vi "Unit Test.vi"() -> ()   [LabVIEW 2019, in "Test.lvlib"]
uses:
  Test.lvlib
  User Event/Controls/UE Abort Action.ctl
  Syringe Pump/NE-500/NE-500.lvlib
  Selection Valve/IDEX/IDEX.lvlib
  LED/LED.lvlib
  IO/sbRIO9623/sbRIO9623.lvlib
  Fluidic Process/Fluidic Process.lvlib
panel:
  in  "UI":bool
  out "Syringe Pump":bool
  out "Selection Valve":bool
  out "LED":bool
  out "I/O":bool
  in  "Open":bool
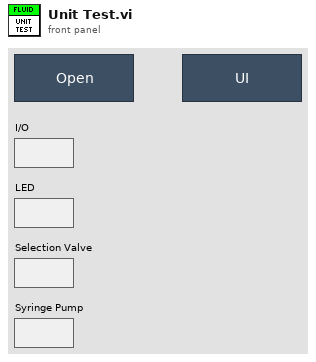
[diagram p1: front panel]
types:
  T1 = typedef "UE Abort Action.ctl" = enum16{"Create", "Get", "Destroy"}
  T2 = typedef "sbRIO9623.lvlib/SEQ Data.ctl" = cluster{"Lid Sensor 1":bool, "Lid Sensor 2":bool, "Laser Interlock":bool, "Buffer Tank":bool, "Wash Tank":bool, "Waste Tank":bool, "SiPM 1":fxp<+,20,5>, "SiPM 2":fxp<+,20,5>, "Initialize Success?":bool, "VI Refnum":refnum<vi>}
  T3 = typedef "LED.lvlib/SEQ Data.ctl" = cluster{"Initialize Sucess?":bool, "BL2 Regulator":dbl, "BL1 Regulator":dbl, "Blood Sensor 1":dbl, "Blood Sensor 2":dbl, "Air Pressure Sensor":dbl, "Force Snesor 1":u32, "Force Snesor 2":u32, "VI Refnum":refnum<vi>}
  T4 = typedef "IDEX.lvlib/SEQ Data.ctl" = cluster{"Position":string, "Initialize Done?":bool, "VI Refnum":refnum<vi>}
  T5 = typedef "NE-500.lvlib/SEQ Data.ctl" = cluster{"Status":string, "Initialize Done?":bool, "VI Refnum":refnum<vi>}
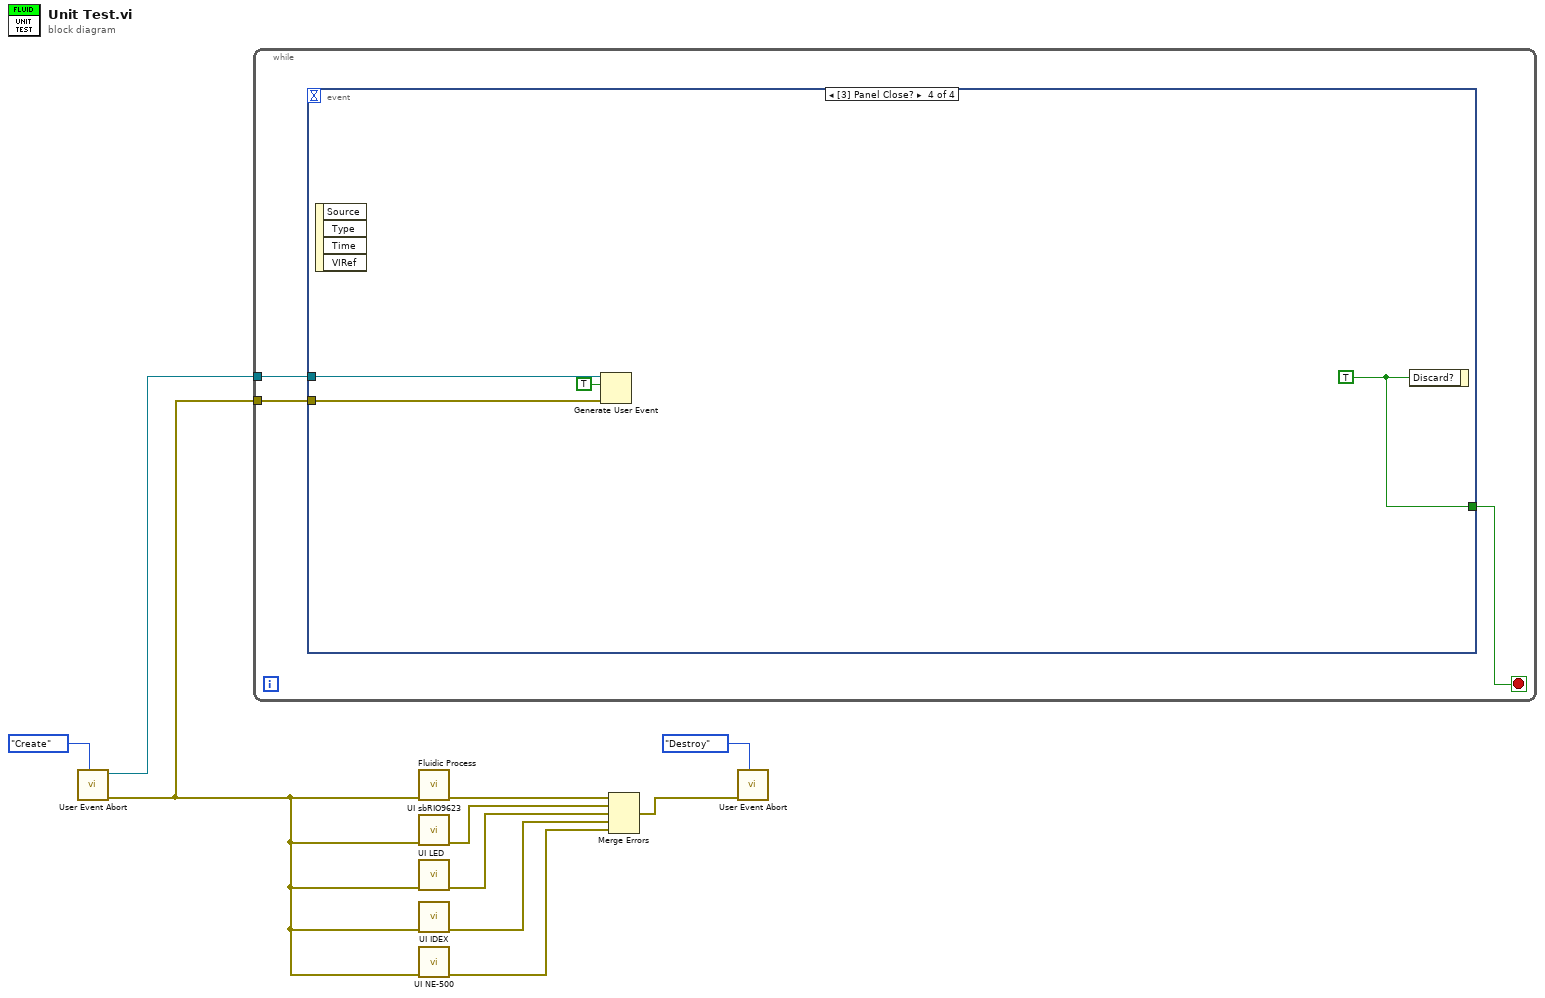
[diagram p0: block diagram]
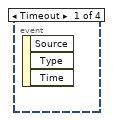
[diagram p2: hidden frame]
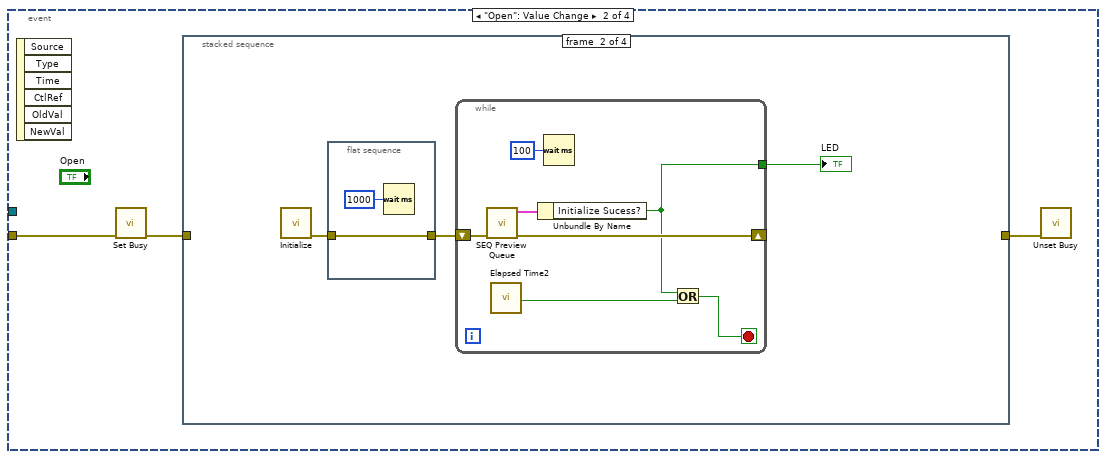
[diagram p3: hidden frame]
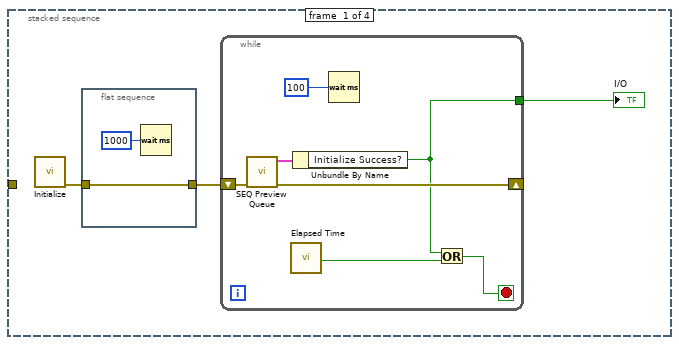
[diagram p4: hidden frame]
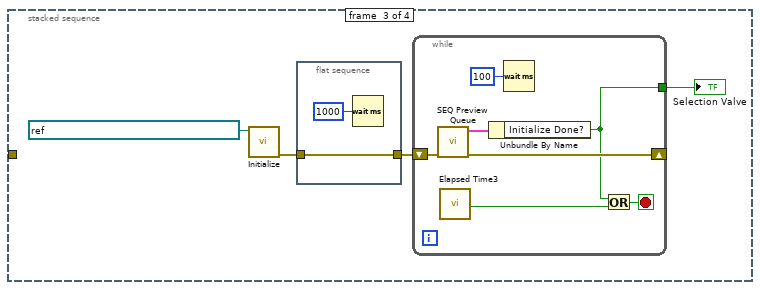
[diagram p5: hidden frame]
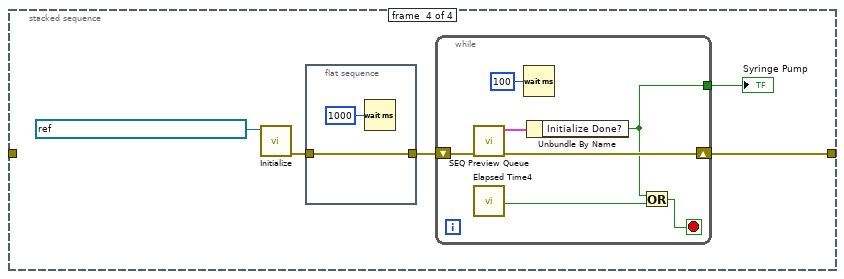
[diagram p6: hidden frame]
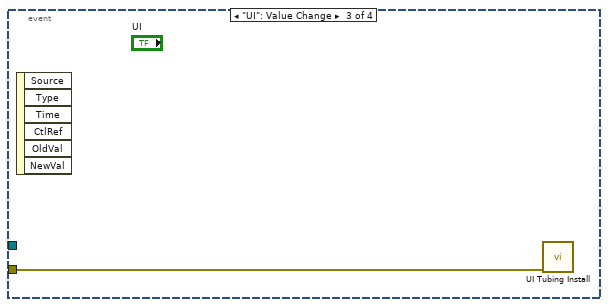
[diagram p7: hidden frame]
diagram:
  n1 = call "User Event Abort.vi"("Action"=UE_Abort_Action."Create") -> ("Error Out"=w1:errorcluster, "User Event Out"=w2:refnum<user-event>)  [unwired: 9 in]
  n2 = while {
    tunnel: w2 -> [w13]
    tunnel: w1 -> [w12]
    stop <- w11 stop-if-true
    n3 = event shown="[3] Panel Close?" {
      selector: _ -> [_ _ _ _]
      dyn-events: _ -> [_ _ _ _]
      timeout: _ -> [_ _ _ _]
      tunnel: w13 -> [_ _ _ w72]
      tunnel: w12 -> [_ w16 w68 w71]
      tunnel: [_ _ _ w69] -> w11
      event Timeout {
        n4 = event-data() -> ()  [unwired: 1 in, 3 out]
      }
      event "Open": Value Change {
        n5 = event-data() -> ()  [unwired: 1 in, 6 out]
        n6 = call <vilib>:"Set Busy.vi"("error in (no error)"=w16) -> ("error out"=w15:errorcluster)  [unwired: 9 in, 1 out]
        n7 = stacked-sequence {
          tunnel: w15 -> [_ _ _ _]
          tunnel: [_ _ _ w56] -> w14
          frame #0 {
            n8 = call "Initialize.vi"() -> ("Error Out"=w19:errorcluster)  [unwired: 11 in]
            n9 = flat-sequence {
              tunnel: w19 -> [w27]
              tunnel: [w27] -> w18
              frame #0 {
                n10 = Wait (ms)(milliseconds to wait=u32 1000) -> ()  [unwired: 1 out]
              }
            }
            n11 = while {
              shift-right: [w25] -> _
              shift-left: w18 -> [w26]
              tunnel: [w21] -> w17
              stop <- w20 stop-if-true
              n12 = call "SEQ Preview Queue.vi"("error in"=w26) -> ("error out"=w25:errorcluster, "SEQ Data"=w24:T2)  [unwired: 9 in]
              n13 = call "Elapsed Time"() -> ("Time has Elapsed"=w23:bool)  [unwired: 12 in, 7 out]
              n14 = Unbundle By Name(w24) -> ("Initialize Success?"=w21:bool)
              n15 = Wait (ms)(milliseconds to wait=u32 100) -> ()  [unwired: 1 out]
              n16 = Or(x=w21, y=w23) -> (x .or. y?=w20:bool)
            }
            "I/O" <- w17
          }
          frame #1 {
            n17 = call "Initialize.vi"() -> ("Error Out"=w31:errorcluster)  [unwired: 11 in]
            n18 = flat-sequence {
              tunnel: w31 -> [w39]
              tunnel: [w39] -> w30
              frame #0 {
                n19 = Wait (ms)(milliseconds to wait=u32 1000) -> ()  [unwired: 1 out]
              }
            }
            n20 = while {
              shift-right: [w36] -> _
              shift-left: w30 -> [w38]
              tunnel: [w33] -> w29
              stop <- w32 stop-if-true
              n21 = call "SEQ Preview Queue.vi"("error in"=w38) -> ("error out"=w36:errorcluster, "SEQ Data"=w35:T3)  [unwired: 9 in]
              n22 = call "Elapsed Time2"() -> ("Time has Elapsed"=w34:bool)  [unwired: 12 in, 7 out]
              n23 = Unbundle By Name(w35) -> ("Initialize Sucess?"=w33:bool)
              n24 = Wait (ms)(milliseconds to wait=u32 100) -> ()  [unwired: 1 out]
              n25 = Or(x=w33, y=w34) -> (x .or. y?=w32:bool)
            }
            "LED" <- w29
          }
          frame #2 {
            n26 = call "Initialize.vi"("VISA name"=refnum<visa-resource-name> "visa://169.254.25.118/ASRL1::INSTR") -> ("Error Out"=w44:errorcluster)  [unwired: 10 in]
            n27 = flat-sequence {
              tunnel: w44 -> [w45]
              tunnel: [w45] -> w43
              frame #0 {
                n28 = Wait (ms)(milliseconds to wait=u32 1000) -> ()  [unwired: 1 out]
              }
            }
            n29 = while {
              tunnel: [w47] -> w42
              shift-right: [w50] -> _
              shift-left: w43 -> [w52]
              stop <- w48 stop-if-true
              n30 = call "SEQ Preview Queue.vi"("error in"=w52) -> ("error out"=w50:errorcluster, "SEQ Data"=w51:T4)  [unwired: 9 in]
              n31 = call "Elapsed Time3"() -> ("Time has Elapsed"=w49:bool)  [unwired: 12 in, 7 out]
              n32 = Unbundle By Name(w51) -> ("Initialize Done?"=w47:bool)
              n33 = Wait (ms)(milliseconds to wait=u32 100) -> ()  [unwired: 1 out]
              n34 = Or(x=w47, y=w49) -> (x .or. y?=w48:bool)
            }
            "Selection Valve" <- w42
          }
          frame #3 {
            n35 = call "Initialize.vi"("VISA name"=refnum<visa-resource-name> "visa://169.254.25.118/ASRL2::INSTR") -> ("Error Out"=w58:errorcluster)  [unwired: 10 in]
            n36 = flat-sequence {
              tunnel: w58 -> [w60]
              tunnel: [w60] -> w57
              frame #0 {
                n37 = Wait (ms)(milliseconds to wait=u32 1000) -> ()  [unwired: 1 out]
              }
            }
            n38 = while {
              shift-right: [w65] -> w56
              shift-left: w57 -> [w67]
              tunnel: [w61] -> w54
              stop <- w62 stop-if-true
              n39 = call "SEQ Preview Queue.vi"("error in"=w67) -> ("error out"=w65:errorcluster, "SEQ Data"=w66:T5)  [unwired: 9 in]
              n40 = call "Elapsed Time4"() -> ("Time has Elapsed"=w63:bool)  [unwired: 12 in, 7 out]
              n41 = Wait (ms)(milliseconds to wait=u32 100) -> ()  [unwired: 1 out]
              n42 = Unbundle By Name(w66) -> ("Initialize Done?"=w61:bool)
              n43 = Or(x=w61, y=w63) -> (x .or. y?=w62:bool)
            }
            "Syringe Pump" <- w54
          }
        }
        n44 = call <vilib>:"Unset Busy.vi"("error in (no error)"=w14) -> ()  [unwired: 10 in, 1 out]
      }
      event "UI": Value Change {
        n45 = event-data() -> ()  [unwired: 1 in, 6 out]
        n46 = call "UI Tubing Install.vi"("error in"=w68) -> ()  [unwired: 10 in, 1 out]
      }
      event Panel Close? {
        w69 = TRUE
        n47 = event-data() -> ()  [unwired: 1 in, 4 out]
        n48 = Generate User Event(user event=w72, event data cluster=TRUE ("event data"), error in=w71) -> ()  [unwired: 1 in, 2 out]
        n49 = event-data("Discard?"=w69) -> ()  [unwired: 1 in, 1 out]
      }
    }
  }
  n50 = call "Fluidic Process.vi"("error in"=w1) -> ("error out"=w8:errorcluster)  [unwired: 10 in]
  n51 = call "UI sbRIO9623.vi"("error in"=w1) -> ("error out"=w6:errorcluster)  [unwired: 10 in]
  n52 = call "UI LED.vi"("error in"=w1) -> ("error out"=w5:errorcluster)  [unwired: 10 in]
  n53 = call "UI IDEX.vi"("error in"=w1) -> ("error out"=w4:errorcluster)  [unwired: 10 in]
  n54 = call "UI NE-500.vi"("error in"=w1) -> ("error out"=w3:errorcluster)  [unwired: 10 in]
  n55 = Merge Errors(w8, w6, w5, w4, w3) -> (w7:errorcluster)
  n56 = call "User Event Abort.vi"("Action"=UE_Abort_Action."Destroy", "Error In"=w7) -> ()  [unwired: 8 in, 2 out]
